vi "Write to File.vi"(8 "error in (no error)":errorcluster, 10 "INI Ref":T1, 11 "Mouse Macro in":refnum<class "Mouse Macro.lvclass">) -> (0 "error out":errorcluster, 2 "INI Ref out":T1, 3 "Mouse Macro out":refnum<class "Mouse Macro.lvclass">)   [LabVIEW 2020, in "MacroAssert.lvlib" / "Mouse Macro.lvclass"]
uses:
  Mouse Macro.lvclass
  Mouse Macro.lvclass/Mouse Macro.ctl
  MacroAssert.lvlib
  <vilib>/Utility/config.llb/NI_LVConfig.lvlib
  <vilib>/Utility/config.llb/Write Key (I32).vi
  <vilib>/Utility/config.llb/Write Key (Boolean).vi
  Macro Step/Macro Step.lvclass
  <vilib>/Utility/config.llb/Config Data RefNum.ctl
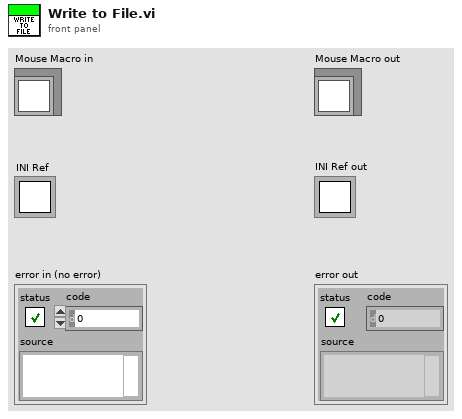
[diagram p1: front panel]
types:
  T1 = typedef "NI_LVConfig.lvlib/Config Data RefNum.ctl" = refnum<k1>
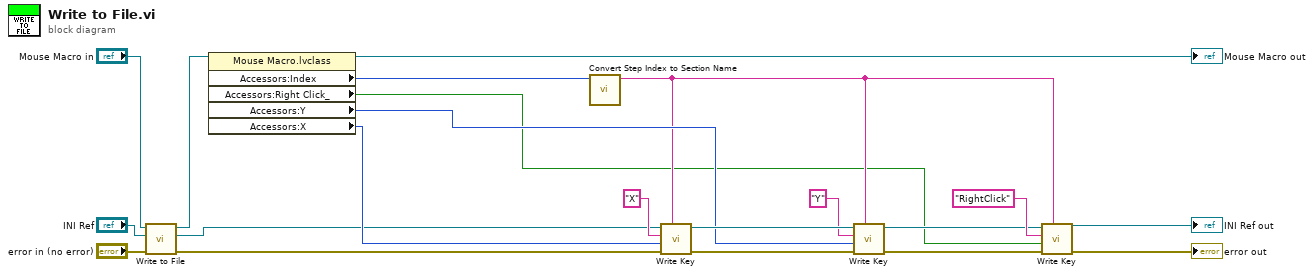
[diagram p0: block diagram]
diagram:
  n1 = call-parent "Write to File.vi"("error in (no error)"="error in (no error)", "INI Ref"="INI Ref", "Macro Step in"="Mouse Macro in") -> ("error out"=w11:errorcluster, "INI Ref out"=w8:T1, "Macro Step out"=w10:refnum<class "Mouse Macro.lvclass">)  [unwired: 6 in]
  n2 = property class="Mouse Macro.lvclass"(reference=w10) -> (reference out=→"Mouse Macro out":refnum<class "Mouse Macro.lvclass">, "Accessors:Index"=w14:i32, "Accessors:Right Click_"=w1:bool, "Accessors:Y"=w12:i32, "Accessors:X"=w13:i32)  [unwired: 1 in, 1 out]
  n3 = call "Convert Step Index to Section Name.vi"("Step Index"=w14) -> ("Section Name"=w2:string)  [unwired: 10 in]
  n4 = call-poly <vilib>:"Write Key.vi"("section"=w2, "error in (no error)"=w11, "value"=w13, "key"="X", "refnum"=w8) -> ("error out"=w16:errorcluster, "refnum out"=w18:T1)  [unwired: 4 in, 1 out]
  n5 = call-poly <vilib>:"Write Key.vi"("section"=w2, "error in (no error)"=w16, "value"=w12, "key"="Y", "refnum"=w18) -> ("error out"=w6:errorcluster, "refnum out"=w5:T1)  [unwired: 4 in, 1 out]
  n6 = call-poly <vilib>:"Write Key.vi"("section"=w2, "error in (no error)"=w6, "value"=w1, "key"="RightClick", "refnum"=w5) -> ("error out"=→"error out":errorcluster, "refnum out"=→"INI Ref out":T1)  [unwired: 4 in, 1 out]
